vi "Read HttpHeaders_Response.vi"(8 "error in (no error)":errorcluster, 11 "HttpResponseMessage in":refnum<class "HttpResponseMessage.lvclass">) -> (0 "error out":errorcluster, 2 "LabVIEWHTTPClient_NET.lvlib:HttpHeaders_Response.lvclass":refnum<class "HttpHeaders_Response.lvclass">, 3 "HttpResponseMessage out":refnum<class "HttpResponseMessage.lvclass">)   [LabVIEW 2018, in "HttpClient_NET.lvlib" / "HttpResponseMessage.lvclass"]
doc: "<b> </b> <b> </b>\nHttpClient_NET\nJustin Young - Viviota\nCopyright (c) 2021\nLicense: BSD"
uses:
  HttpResponseMessage.lvclass
  HttpHeaders_response/HttpHeaders_Response.lvclass
  HttpResponseMessage.lvclass/HttpResponseMessage.ctl
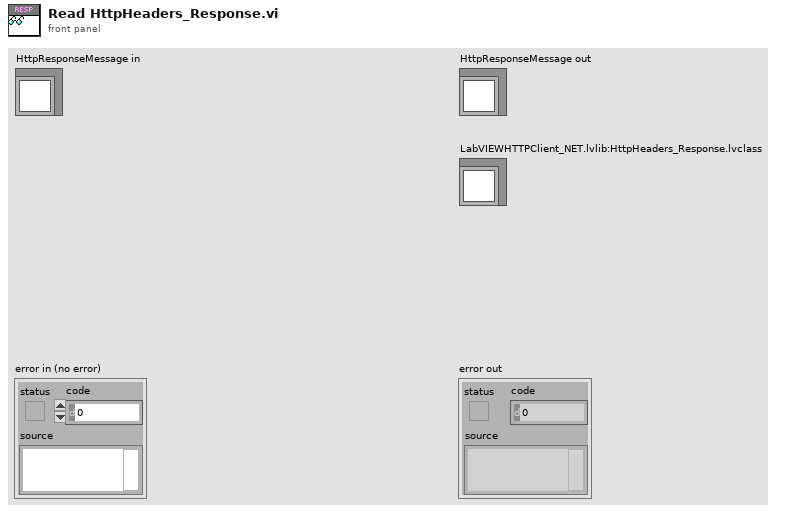
[diagram p1: front panel]
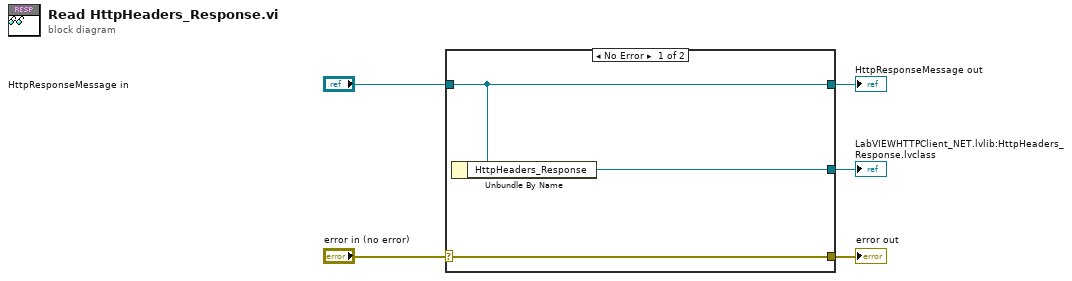
[diagram p0: block diagram]
diagram:
  n1 = case shown="No Error" "error in (no error)" {
    selector: "error in (no error)" -> [w8 w9]
    tunnel: [w8 w9] -> w4
    tunnel: [w7 w10] -> w2
    tunnel: "HttpResponseMessage in" -> [w7 w10]
    tunnel: [w6 _] -> w1
    frame No Error {
      n2 = Unbundle By Name(w7) -> ("HttpHeaders_Response"=w6:refnum<class "HttpHeaders_Response.lvclass">)
    }
    frame Error {
    }
  }
  "error out" <- w4
  "HttpResponseMessage out" <- w2
  "LabVIEWHTTPClient_NET.lvlib:HttpHeaders_Response.lvclass" <- w1
